vi "Set Indexed Waveform Chart Plot Names.vi"(8 "error in (no error)":errorcluster, 9 "Indices":u32[](array[numeric]), 10 "Plot Names":string[](array[string]), 11 "reference in":refnum<vi>) -> (0 "error out":errorcluster, 3 "reference out":refnum<vi>)   [LabVIEW 2018]
doc: "Sets the indexed plot names in a waveform chart legend and makes the plot visible. If the index is larger than the minimum number of plots property of the waveform chart, this property is modified to allow the name to be assigned without error. Supports any waveform chart type."
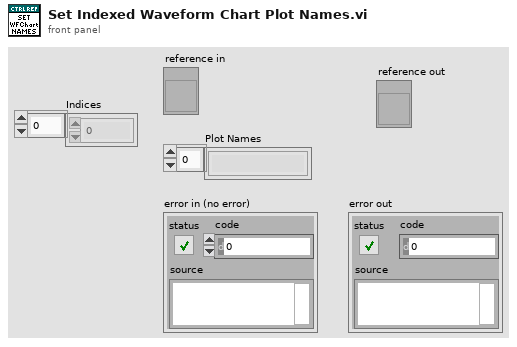
[diagram p1: front panel]
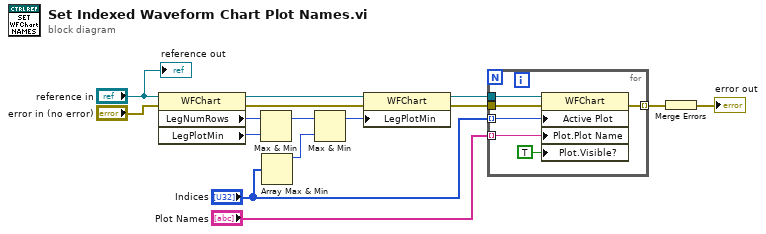
[diagram p0: block diagram]
diagram:
  n1 = property on="Property Node" class="WFChart"(reference="reference in", error in="error in (no error)") -> (reference out=w10:refnum<vi>, error out=w7:errorcluster, "LegNumRows"=w12:u32, "LegPlotMin"=w11:u32)
  n2 = Max & Min(x=w12, y=w11) -> (max(x,y)=w6:u32)  [unwired: 1 out]
  n3 = Array Max & Min(array="Indices") -> (max value=w5:u32)  [unwired: 3 out]
  n4 = Max & Min(x=w6, y=w5) -> (max(x,y)=w4:u32)  [unwired: 1 out]
  n5 = property on="Property Node" class="WFChart"(reference=w10, error in=w7, "LegPlotMin"=w4) -> (reference out=w9:refnum<vi>, error out=w8:errorcluster)
  n6 = for {
    tunnel: [w21] -> w14 mode=indexing
    tunnel: w9 -> [w20]
    tunnel: w8 -> [w19]
    tunnel: "Indices" -> [w18] mode=indexing
    tunnel: "Plot Names" -> [w17] mode=indexing
    n7 = property on="Property Node" class="WFChart"(reference=w20, error in=w19, "Active Plot"=w18, "Plot.Plot Name"=w17, "Plot.Visible?"=TRUE ("Plot.Visible")) -> (error out=w21:errorcluster)  [unwired: 1 out]
  }
  n8 = Merge Errors(w14) -> (→"error out":errorcluster)
  "reference out" <- "reference in"
